vi "readClearErrorIsTrueSV.vi"(8 "error in (no error)":errorcluster, 11 "ApplicationHandler in":refnum<class "ApplicationHandler.lvclass">) -> (0 "error out":errorcluster, 2 "ClearErrorIsTrue":bool, 3 "ApplicationHandler out":refnum<class "ApplicationHandler.lvclass">)   [LabVIEW 2013, in "ComponentData.lvlib" / "ApplicationHandler.lvclass"]
uses:
  <userlib>/Common/Component/common_application/RT/ComponentData/ApplicationHandler/ApplicationHandler.lvclass
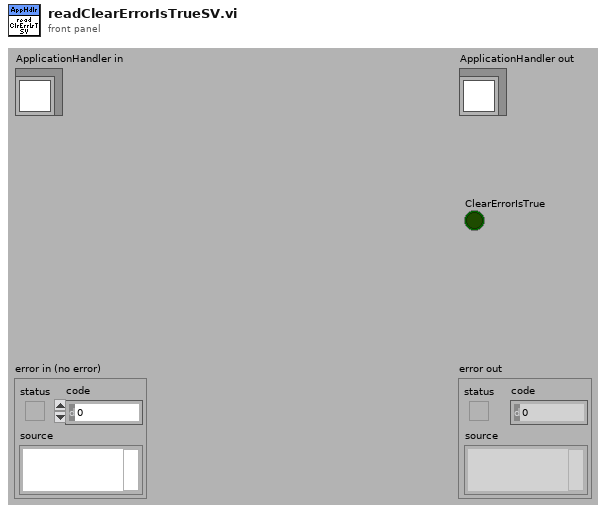
[diagram p1: front panel]
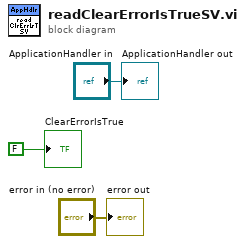
[diagram p0: block diagram]
diagram:
  "error out" <- "error in (no error)"
  "ApplicationHandler out" <- "ApplicationHandler in"
  "ClearErrorIsTrue" <- FALSE
